vi "Get Wavelength or frequency.vi"(8 "error in (no error)":errorcluster, 9 "air or vac (air)":enum16{"air", "vac"}(ring), 10 "mode (wavelength)":enum16{"wavelength (nm)", "frequency (THz)"}(ring), 11 "Quiet Errors?":bool) -> (0 "error out":errorcluster, 2 "result":dbl)   [LabVIEW 2009]
doc: "Gets the current wavelenth (nm) or frequency (THz) from the wavelength meter. Maximum repetition rate appears to be 0.03 ms per reading (~30 kHz).\n\nSet QuietErrors? to True for use with scans or etches, then handle errors externally."
uses:
  <vilib>/Utility/error.llb/DialogType.ctl
  WINDOWS/system32/wlmData.dll
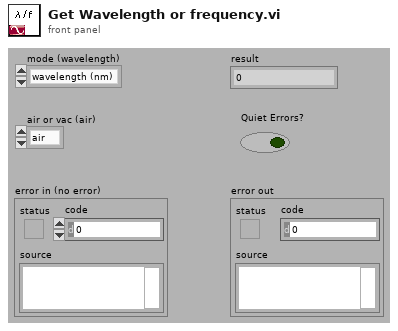
[diagram p1: front panel]
types:
  T1 = typedef "DialogType.ctl" = u16
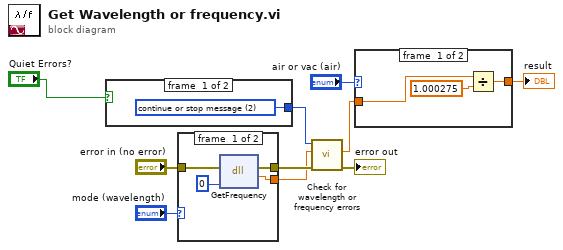
[diagram p0: block diagram]
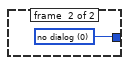
[diagram p2: hidden frame]
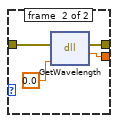
[diagram p3: hidden frame]
diagram:
  n1 = case shown="False" "Quiet Errors?" {
    tunnel: [w11 w12] -> w2
    frame #0 {
      w11 = T1 2 items=["no dialog", "OK message", "continue or stop message", "OK message + warnings", "continue/stop + warnings"] ("type of dialog")
    }
    frame #1 {
      w12 = T1 0 items=["no dialog", "OK message", "continue or stop message", "OK message + warnings", "continue/stop + warnings"] ("type of dialog")
    }
  }
  n2 = case shown="\"wavelength (nm)\", Default" "mode (wavelength)" {
    tunnel: "error in (no error)" -> [w15 w19]
    tunnel: [w14 w18] -> w9
    tunnel: [w13 w17] -> w8
    frame #0 {
      n3 = dll-call lib="C:/WINDOWS/system32/wlmData.dll" fn="GetFrequency"(error in=w15, "F"=0) -> (error out=w14:errorcluster, "return type"=w13:dbl)  [unwired: 3 in, 1 out]
    }
    frame #1 {
      n4 = dll-call lib="C:/WINDOWS/system32/wlmData.dll" fn="GetWavelength"(error in=w19, "WL"=0.0 ("F")) -> (error out=w18:errorcluster, "return type"=w17:dbl)  [unwired: 3 in, 1 out]
    }
  }
  n5 = call "Check for wavelength or frequency errors.vi"("error in (no error)"=w9, "F or lambda in"=w8, "type of dialog"=w2) -> ("error out"=→"error out":errorcluster, "F or lambda out"=w5:dbl)  [unwired: 7 out]
  n6 = case shown="\"air\", Default" "air or vac (air)" {
    tunnel: w5 -> [w23 w24]
    tunnel: [w21 w24] -> w4
    frame #0 {
      n7 = Divide(x=w23, y=1.000275) -> (x/y=w21:dbl)
    }
    frame #1 {
    }
  }
  "result" <- w4
